vi "Robot Global Data.vi"() -> ()   [LabVIEW 2017]
doc: "This global VI can contain as many global variables as you need. Place a control on the panel, give it a good name. To read or write to it from a VI, drag the icon to the diagram of that VI. You can also drag from the project. Click on the node to change which global you access. You shouldn't have multiple locations writing to a global or it will cause a race-condition."
uses:
  <vilib>/Rock Robotics/WPI/Camera/WPI_CameraImageSize.ctl
  <vilib>/Rock Robotics/WPI/DriverStation/WPI_DriverStationRobotMode2.ctl
panel:
  out "Auto Angle Right Drive":dbl
  out "Auto Angle Left Drive":dbl
  in  "Right Encoder Pos":dbl
  in  "Left Encoder Pos":dbl
  out "Joystick 0 Button 9":bool
  out "PushCubeFromAuton":bool
  out "RaiseShooterAuton":bool
  in  "Gyro":dbl
  out "Auto Shooter":dbl
  out "Auto Intake Speed":dbl
  out "Auto Distance Right Drive":dbl
  out "Auto Distance Left Drive":dbl
  in  "ShootCancel":dbl
  out "SwitchIntakeSpeed":dbl
  out "PushCubeFromSwitch":bool
  out "IntakeIntakeSpeed":dbl
  out "PushCubeFromScale":bool
  out "RaiseShooterfromScale":bool
  out "SwitchShooterSpeed":dbl
  out "ScaleShooterSpeed":dbl
  out "Joystick 1 Button 4":bool
  out "Joystick 1 Button 5":bool
  in  "Joystick 0 Axis 4":dbl
  in  "Joystick 0 Axis 1":dbl
  in  "Robot Mode":T1
  in  "image size":T2=enum."320x240"
  in  "Enable Vision":bool
  # "Joysticks"
  # "Sensors"
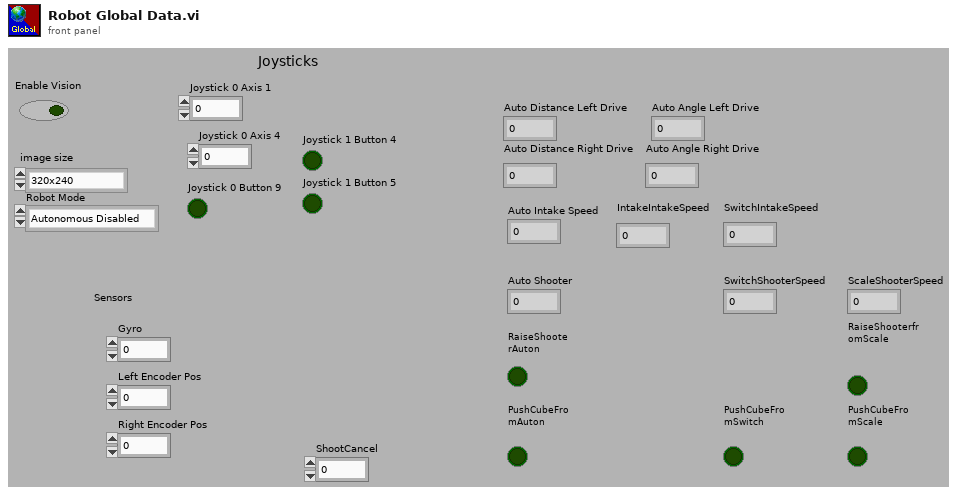
[diagram p1: front panel]
types:
  T1 = typedef "WPI_DriverStationRobotMode2.ctl" = enum16{"Autonomous Disabled", "Autonomous Enabled", "Teleop Disabled", "Teleop Enabled", "Disconnected", "Finish", "Test Disabled", "Test Enabled", "Emergency Stopped"}
  T2 = typedef "WPI_CameraImageSize.ctl" = enum16{"640x480", "320x240", "160x120", "Custom"}
diagram:
